vi "Calibration_ver1.vi"() -> ()   [LabVIEW 2018]
uses:
  <vilib>/Utility/file.llb/Write Delimited Spreadsheet (DBL).vi
panel:
  out "Current Status":string
  out "XY Graph":cluster{"InputArray":dbl[], dbl[]}[](graph)
  out "Outputs":dbl[][](array[numeric])
  in  "SamplingRate(Hz)":dbl=2000.0 format="%0.2f"
  in  "InputArray":dbl[](array[numeric])=[0.2, 0.4, 0.6, 0.8, 1.0, 1.5, 2.0, 2.5, 3.0, 3.5, 4.0, 5.0]
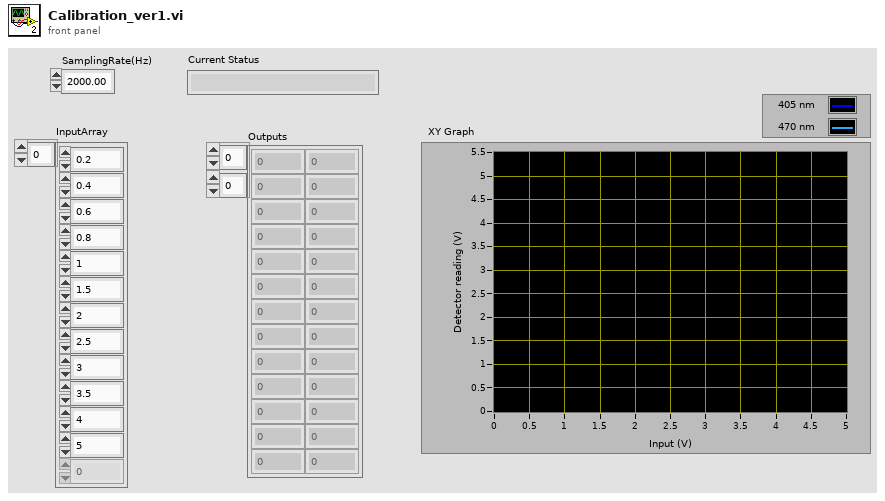
[diagram p1: front panel]
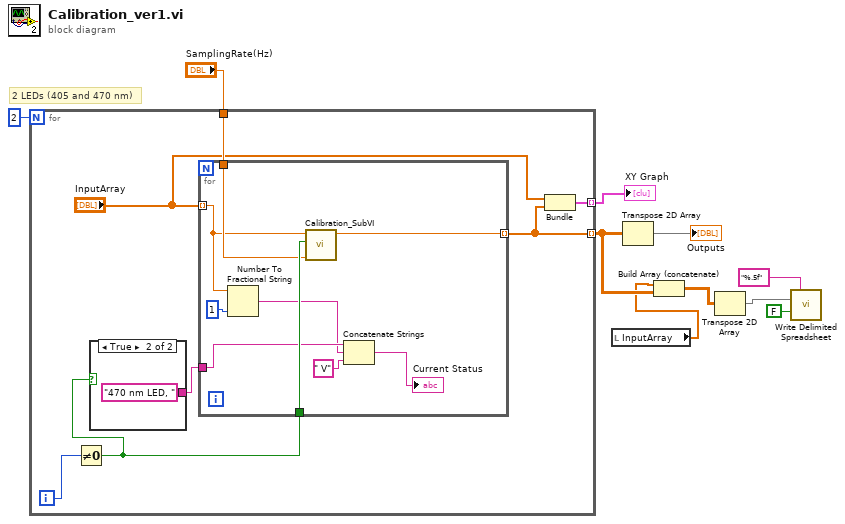
[diagram p0: block diagram]
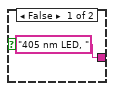
[diagram p2: hidden frame]
diagram:
  # "2 LEDs (405 and 470 nm)"
  n1 = for {
    N: 2 -> [_]
    tunnel: "SamplingRate(Hz)" -> [w16]
    tunnel: [w15] -> w4 mode=indexing
    tunnel: [w13] -> w8 mode=indexing
    i -> [w17]
    n2 = Not Equal To 0?(x=w17) -> (x != 0?=w12:bool)
    n3 = case shown="True" w12 {
      tunnel: ["405 nm LED, " "470 nm LED, "] -> w11
      frame False {
      }
      frame True {
      }
    }
    n4 = for {
      tunnel: "InputArray" -> [w25] mode=indexing
      tunnel: w12 -> [w28]
      tunnel: w16 -> [w27]
      tunnel: [w26] -> w15 mode=indexing
      tunnel: w11 -> [w24]
      n5 = Number To Fractional String(number=w25, precision (6)=i16 1 ("width (-)")) -> (F-format string=w23:string)  [unwired: 2 in]
      n6 = call "Calibration_SubVI.vi"("SamplingRate(Hz)"=w27, "LED"=w28, "Input (V)"=w25) -> ("mean"=w26:dbl)  [unwired: 8 in]
      n7 = Concatenate Strings(w24, w23, " V") -> (→"Current Status":string)
    }
    n8 = Bundle("InputArray"="InputArray", w15) -> (w13:cluster{"InputArray":dbl[], dbl[]})  [unwired: 1 in]
  }
  "XY Graph" <- w8
  n9 = local read "InputArray"() -> (w3:dbl[])
  n10 = Transpose 2D Array(2D array=w4) -> (transposed array=→"Outputs":dbl[][])
  n11 = Build Array (concatenate)(w3, w4) -> (w2:dbl[][])
  n12 = Transpose 2D Array(2D array=w2) -> (transposed array=w1:dbl[][])
  n13 = call-poly <vilib>:"Write Delimited Spreadsheet.vi"("format (%.3f)"="%.5f", "2D data"=w1, "append to file? (new file:F)"=FALSE) -> ()  [unwired: 11 in, 2 out]
